vi "step4.vi"(1 "NT":u32, 2 "C1":bool, 3 "NC1":u32, 4 "C2":bool, 5 "NC2":u32, 6 "C3":bool, 7 "NC3":u32, 8 "T":u32, 9 "C4":bool, 11 "NC4":u32, 16 "N step":u32) -> (19 "N step out":u32, 20 "T NT":u32[](array[numeric]), 21 "C NC":cluster{"C":bool, "NC":u32}[](array[cluster]))   [LabVIEW 2019, in "Userlib.lvlib"]
uses:
  Userlib.lvlib
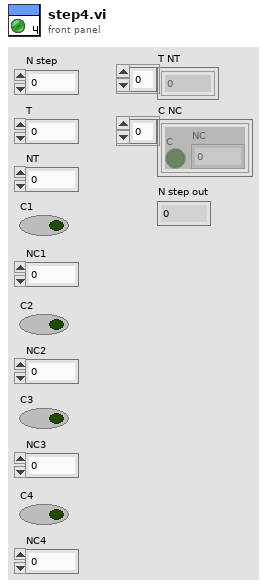
[diagram p1: front panel]
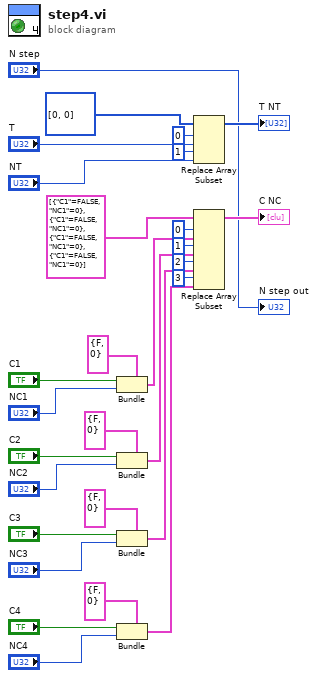
[diagram p0: block diagram]
diagram:
  n1 = Bundle(cluster=cluster{"C1":bool, "NC1":u32} {"C1"=FALSE, "NC1"=0}, "C1"="C1", "NC1"="NC1") -> (w18:cluster{"C1":bool, "NC1":u32})
  n2 = Bundle(cluster=cluster{"C1":bool, "NC1":u32} {"C1"=FALSE, "NC1"=0}, "C1"="C2", "NC1"="NC2") -> (w12:cluster{"C1":bool, "NC1":u32})
  n3 = Bundle(cluster=cluster{"C1":bool, "NC1":u32} {"C1"=FALSE, "NC1"=0}, "C1"="C3", "NC1"="NC3") -> (w7:cluster{"C1":bool, "NC1":u32})
  n4 = Bundle(cluster=cluster{"C1":bool, "NC1":u32} {"C1"=FALSE, "NC1"=0}, "C1"="C4", "NC1"="NC4") -> (w1:cluster{"C1":bool, "NC1":u32})
  n5 = Replace Array Subset(array=u32[] [0, 0] ("appended array"), new element #1="T", index #1=0 ("index"), new element #2="NT", index #2=1 ("index")) -> (→"T NT":u32[])
  n6 = Replace Array Subset(array=cluster{"C1":bool, "NC1":u32}[] [{"C1"=FALSE, "NC1"=0}, {"C1"=FALSE, "NC1"=0}, {"C1"=FALSE, "NC1"=0}, {"C1"=FALSE, "NC1"=0}] ("appended array"), new element #1=w18, index #1=0 ("index"), new element #2=w12, index #2=1 ("index"), new element #3=w7, index #3=2 ("index"), new element #4=w1, index #4=3 ("index")) -> (→"C NC":cluster{"C1":bool, "NC1":u32}[])
  "N step out" <- "N step"
